vi "poly_cast_variant_U8.vi"(2 "variant":variant) -> (7 "data (255)":u8)   [LabVIEW 2015]
doc: "This vi attempts to cast a variant to data. The data is set to default value if an error occurs. This vi is intended to be used as a convenience tool when the data type is unambigous.\n\nWritten by Marcin Konowalczyk\nTimmel Group @ Oxford University"
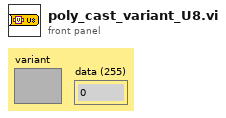
[diagram p1: front panel]
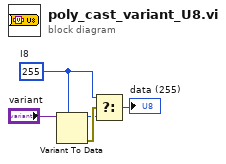
[diagram p0: block diagram]
diagram:
  w3 = u8 255  # I8
  n1 = Variant To Data(type=w3, Variant="variant") -> (data=w1:u8, error out=w4:errorcluster)  [unwired: 1 in]
  n2 = Select(t=w3, s=w4, f=w1) -> (s? t:f=→"data (255)":u8)
